vi "read_Ga.vi"() -> (0 "H2 Dilute":bool, 1 "GAMFC3":dbl, 2 "GAMFC2":dbl, 3 "GAMFC1":dbl, 4 "Remote":bool, 5 "Run":bool, 6 "Bubbler In":bool, 7 "Active":bool)   [LabVIEW 2011]
uses:
  low_level_proc/globals.vi
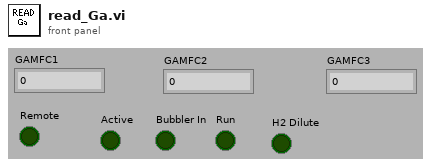
[diagram p1: front panel]
types:
  T1 = typedef "relaySpec.ctl" = cluster{"Card Index":u16, "Relay Index":u16}
  T2 = typedef "DA_Spec.ctl" = cluster{"Card Index":u16, "Channel Index":u16}
  T3 = typedef "AD_Spec.ctl" = u16
  T4 = cluster{"Relay Functions":cluster{"Remote":T1, "Active":T1, "Bubbler In":T1, "H2 dilute":T1, "Run":T1}, "D/A Functions":cluster{"Flow 1":T2, "Flow 2":T2, "Flow 3":T2}, "Flow Ranges":cluster{"Flow 1 (GAMFC1)":u16, "Flow 2 (GAMFC2)":u16, "Flow 3 (GAMFC3)":u16}, "A/D Functions":cluster{"Flow 1":T3, "Flow 2":T3, "Flow 3":T3}}
  T5 = cluster{"Remote":T1, "Active":T1, "Bubbler In":T1, "H2 dilute":T1, "Run":T1}
  T6 = cluster{"Flow 1 (GAMFC1)":u16, "Flow 2 (GAMFC2)":u16, "Flow 3 (GAMFC3)":u16}
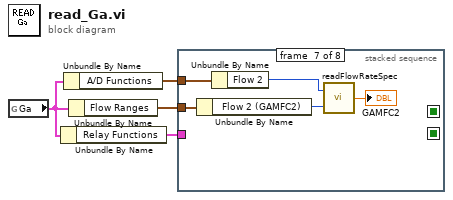
[diagram p0: block diagram]
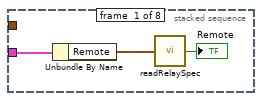
[diagram p2: hidden frame]
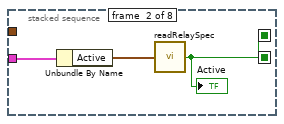
[diagram p3: hidden frame]
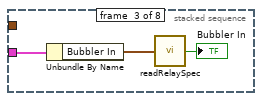
[diagram p4: hidden frame]
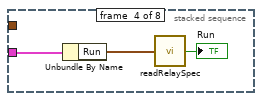
[diagram p5: hidden frame]
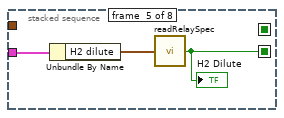
[diagram p6: hidden frame]
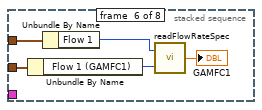
[diagram p7: hidden frame]
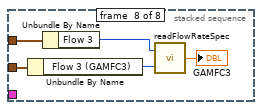
[diagram p8: hidden frame]
diagram:
  n1 = global read "globals.vi" "Ga"() -> (w3:T4)
  n2 = Unbundle By Name(w3) -> ("Relay Functions"=w4:T5)
  n3 = Unbundle By Name(w3) -> ("A/D Functions"=w2:cluster{"Flow 1":T3, "Flow 2":T3, "Flow 3":T3})
  n4 = Unbundle By Name(w3) -> ("Flow Ranges"=w1:T6)
  n5 = stacked-sequence {
    seq-local: [_ w10 _ _ _ _ _ _] -> [_ _ _ _ _ _ _ _]
    seq-local: [_ _ _ _ w19 _ _ _] -> [_ _ _ _ _ _ _ _]
    tunnel: w4 -> [w6 w9 w12 w15 w18 _ _ _]
    tunnel: w2 -> [_ _ _ _ _ w24 w26 w31]
    tunnel: w1 -> [_ _ _ _ _ w21 w25 w33]
    frame #0 {
      n6 = Unbundle By Name(w6) -> ("Remote"=w5:T1)
      n7 = call "readRelaySpec.vi"("RelaySpec"=w5) -> ("Relay Status"=→"Remote":bool)
    }
    frame #1 {
      n8 = Unbundle By Name(w9) -> ("Active"=w8:T1)
      n9 = call "readRelaySpec.vi"("RelaySpec"=w8) -> ("Relay Status"=w10:bool)
      "Active" <- w10
    }
    frame #2 {
      n10 = Unbundle By Name(w12) -> ("Bubbler In"=w11:T1)
      n11 = call "readRelaySpec.vi"("RelaySpec"=w11) -> ("Relay Status"=→"Bubbler In":bool)
    }
    frame #3 {
      n12 = Unbundle By Name(w15) -> ("Run"=w14:T1)
      n13 = call "readRelaySpec.vi"("RelaySpec"=w14) -> ("Relay Status"=→"Run":bool)
    }
    frame #4 {
      n14 = Unbundle By Name(w18) -> ("H2 dilute"=w17:T1)
      n15 = call "readRelaySpec.vi"("RelaySpec"=w17) -> ("Relay Status"=w19:bool)
      "H2 Dilute" <- w19
    }
    frame #5 {
      n16 = Unbundle By Name(w21) -> ("Flow 1 (GAMFC1)"=w20:u16)
      n17 = Unbundle By Name(w24) -> ("Flow 1"=w22:T3)
      n18 = call "readFlowRateSpec.vi"("Flow range Index"=w20, "Channel Index"=w22) -> ("Flow Rate (sccm)"=→"GAMFC1":dbl)
    }
    frame #6 {
      n19 = Unbundle By Name(w25) -> ("Flow 2 (GAMFC2)"=w28:u16)
      n20 = Unbundle By Name(w26) -> ("Flow 2"=w29:T3)
      n21 = call "readFlowRateSpec.vi"("Flow range Index"=w28, "Channel Index"=w29) -> ("Flow Rate (sccm)"=→"GAMFC2":dbl)
    }
    frame #7 {
      n22 = Unbundle By Name(w33) -> ("Flow 3 (GAMFC3)"=w32:u16)
      n23 = Unbundle By Name(w31) -> ("Flow 3"=w30:T3)
      n24 = call "readFlowRateSpec.vi"("Flow range Index"=w32, "Channel Index"=w30) -> ("Flow Rate (sccm)"=→"GAMFC3":dbl)
    }
  }
